vi "CalCurrent.vi"(0 "AD1":u64, 1 "AD2":u64, 2 "REAL1":dbl, 3 "REAL2":dbl, 8 "类型":u32(ring)=4 items=["PCI5121"=1, "PCI9810"=2, "USBCAN1"=3, "USBCAN2"=4, "PCI9820"=5, "CAN232"=6, "PCI5110"=7, "CANLite(mini)"=8, "ISA9620"=9, "ISA5420"=10, "PC104CAN"=11, "CANET"=17, "DNP9810"=13, "USBCAN-E-U"=20, "USBCAN-2E-U"=21], 10 "设备索引":u32(ring) items=["0", "1", "2", "3", "4", "5", "6", "7", "8", "9", "10", "11", "12", "13", "14", "15", ""], 12 "CAN路数":u32(ring) items=["0", "1"], 14 "ExternFlag":u8, 16 "ID Send":u32, 18 "DataLen":u8) -> (20 "发送状态":bool, 21 "Gain":dbl)   [LabVIEW 2013]
uses:
  BHN01/AutoBurn/Settings/ControlCAN.dll
panel:
  in  "设备索引 2":u32(ring) items=["0", "1", "2", "3", "4", "5", "6", "7", "8", "9", "10", "11", "12", "13", "14", "15", ""]
  in  "CAN路数 2":u32(ring) items=["0", "1"]
  in  "类型 2":u32(ring)=4 items=["PCI5121"=1, "PCI9810"=2, "USBCAN1"=3, "USBCAN2"=4, "PCI9820"=5, "CAN232"=6, "PCI5110"=7, "CANLite(mini)"=8, "ISA9620"=9, "ISA5420"=10, "PC104CAN"=11, "CANET"=17, "DNP9810"=13, "USBCAN-E-U"=20, "USBCAN-2E-U"=21]
  out "VCI_CAN_OBJ_T":T1 {"ID" format="%x"}
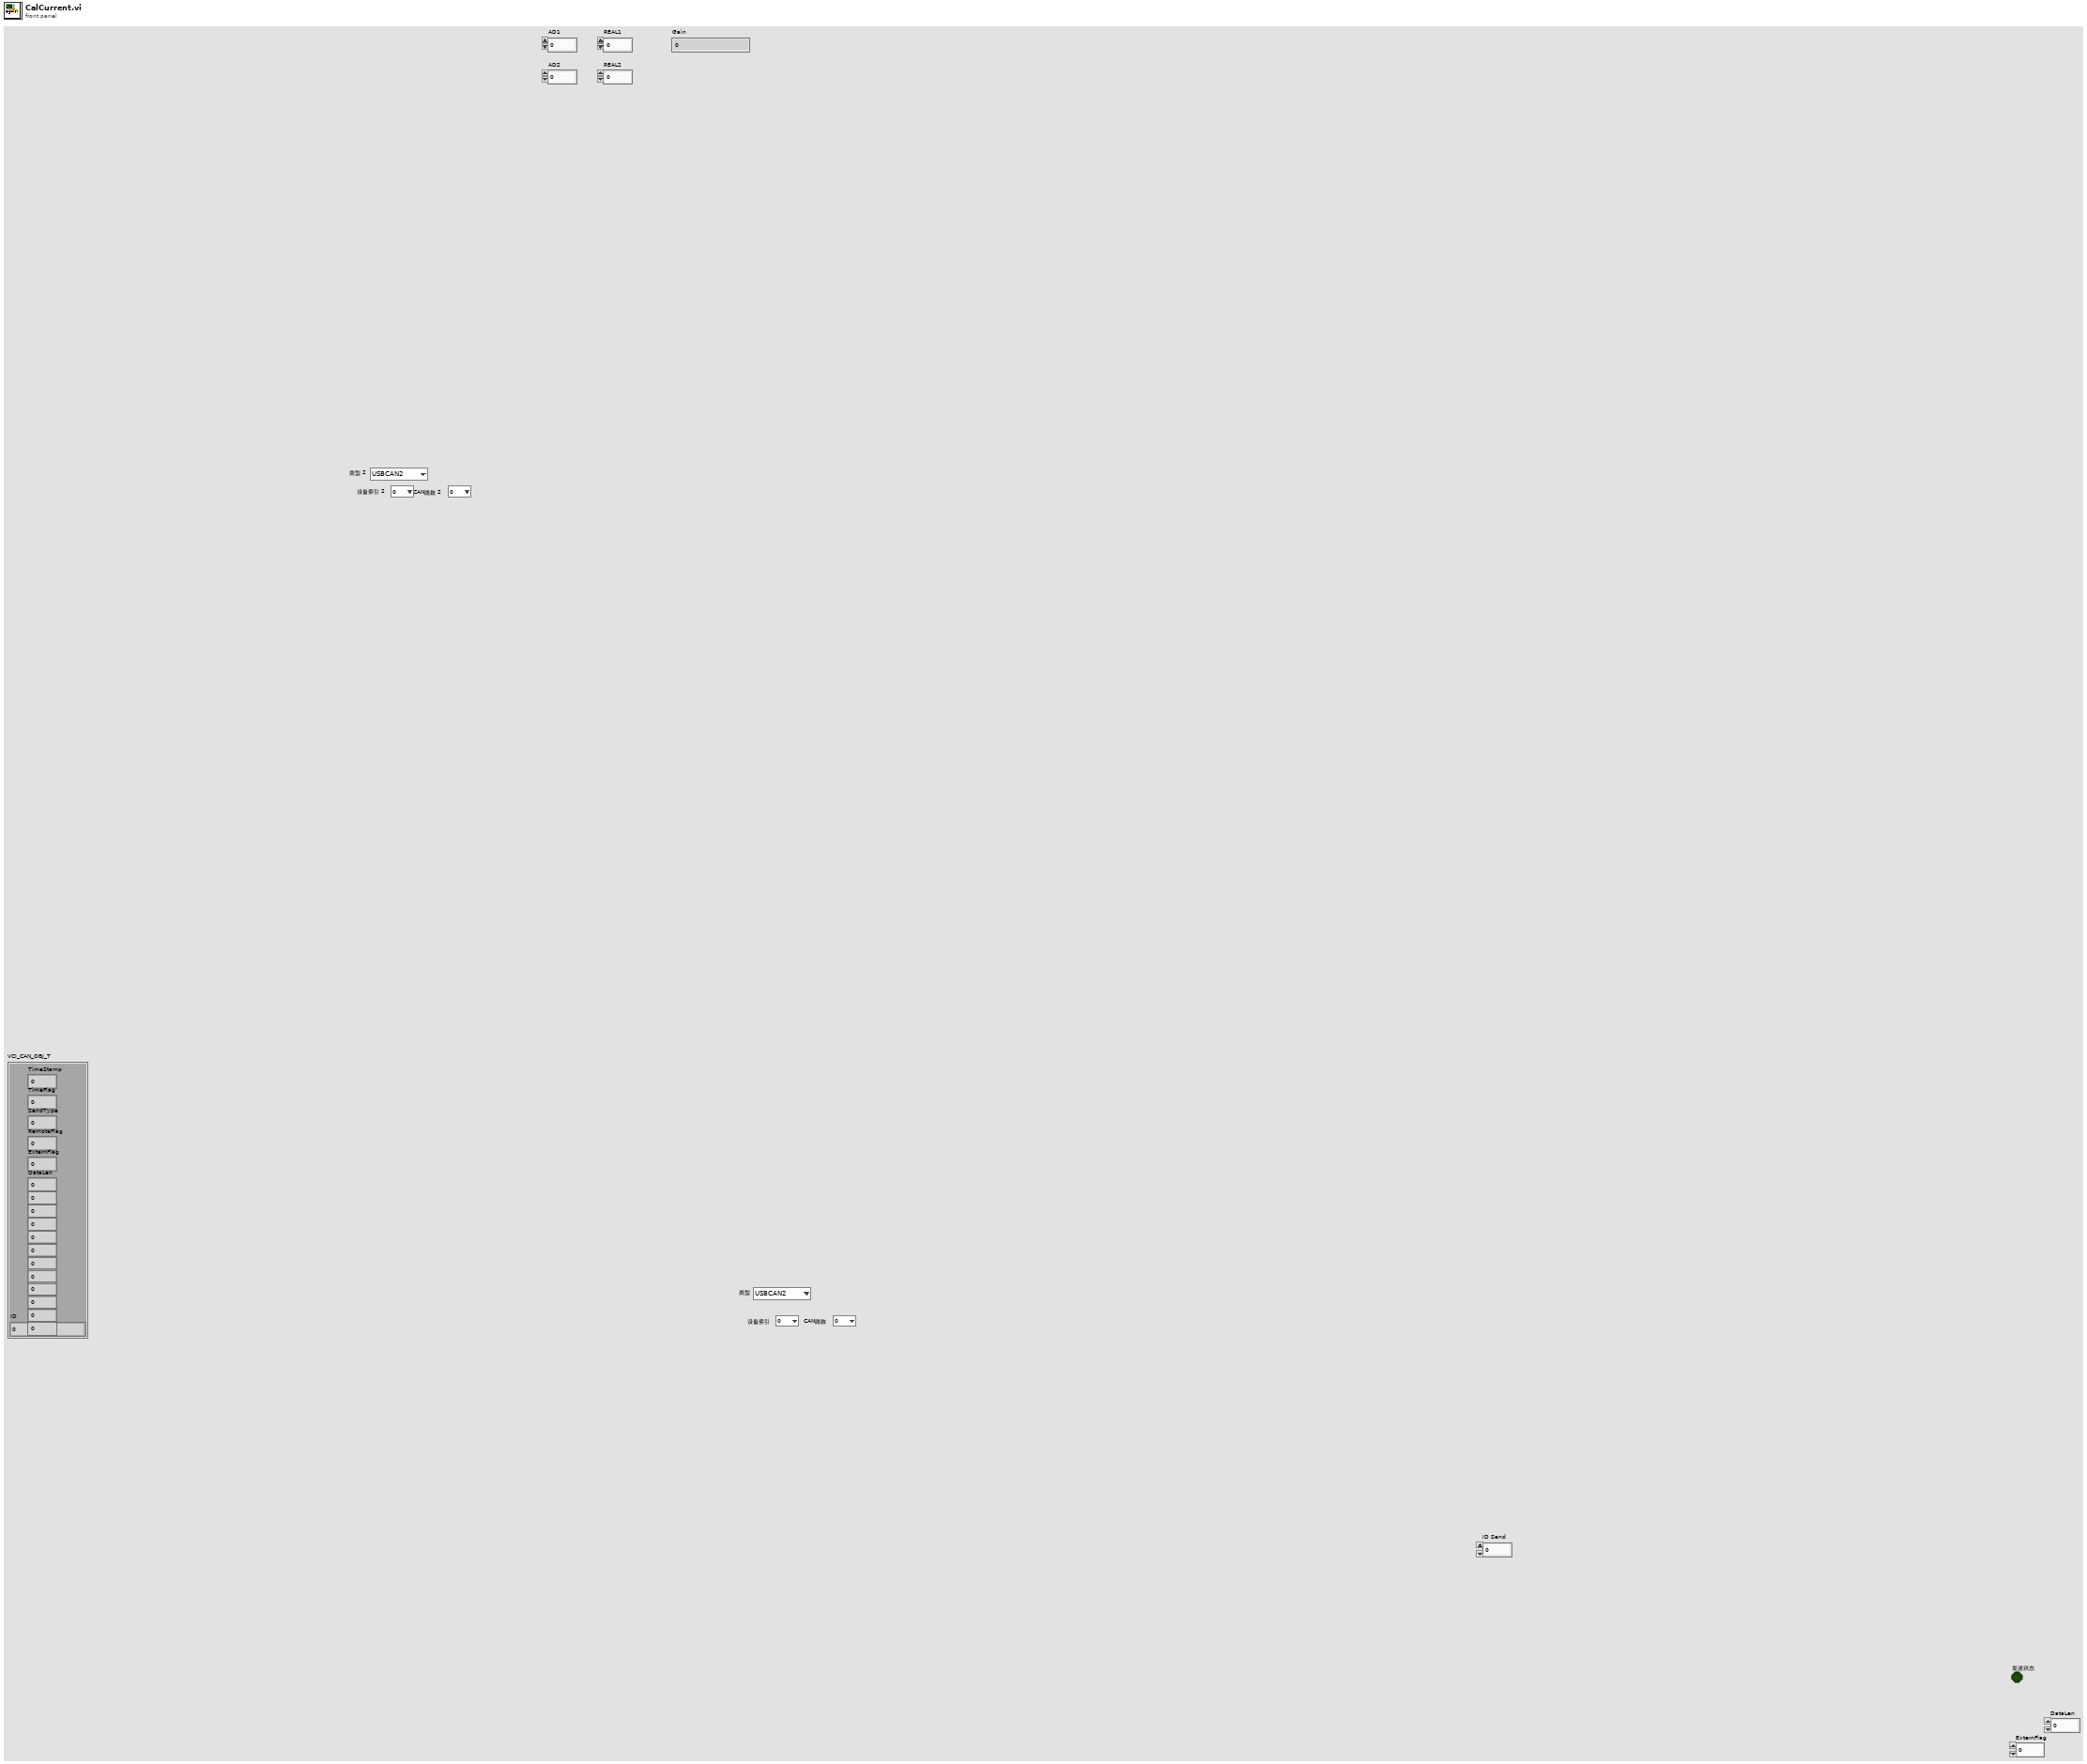
[diagram p1: front panel]
types:
  T1 = cluster{"ID":u32, "TimeStamp":u32, "TimeFlag":u8, "SendType":u8, "RemoteFlag":u8, "ExternFlag":u8, "DataLen":u8, u8, u8, u8, u8, u8, u8, u8, u8, u8, u8, u8}
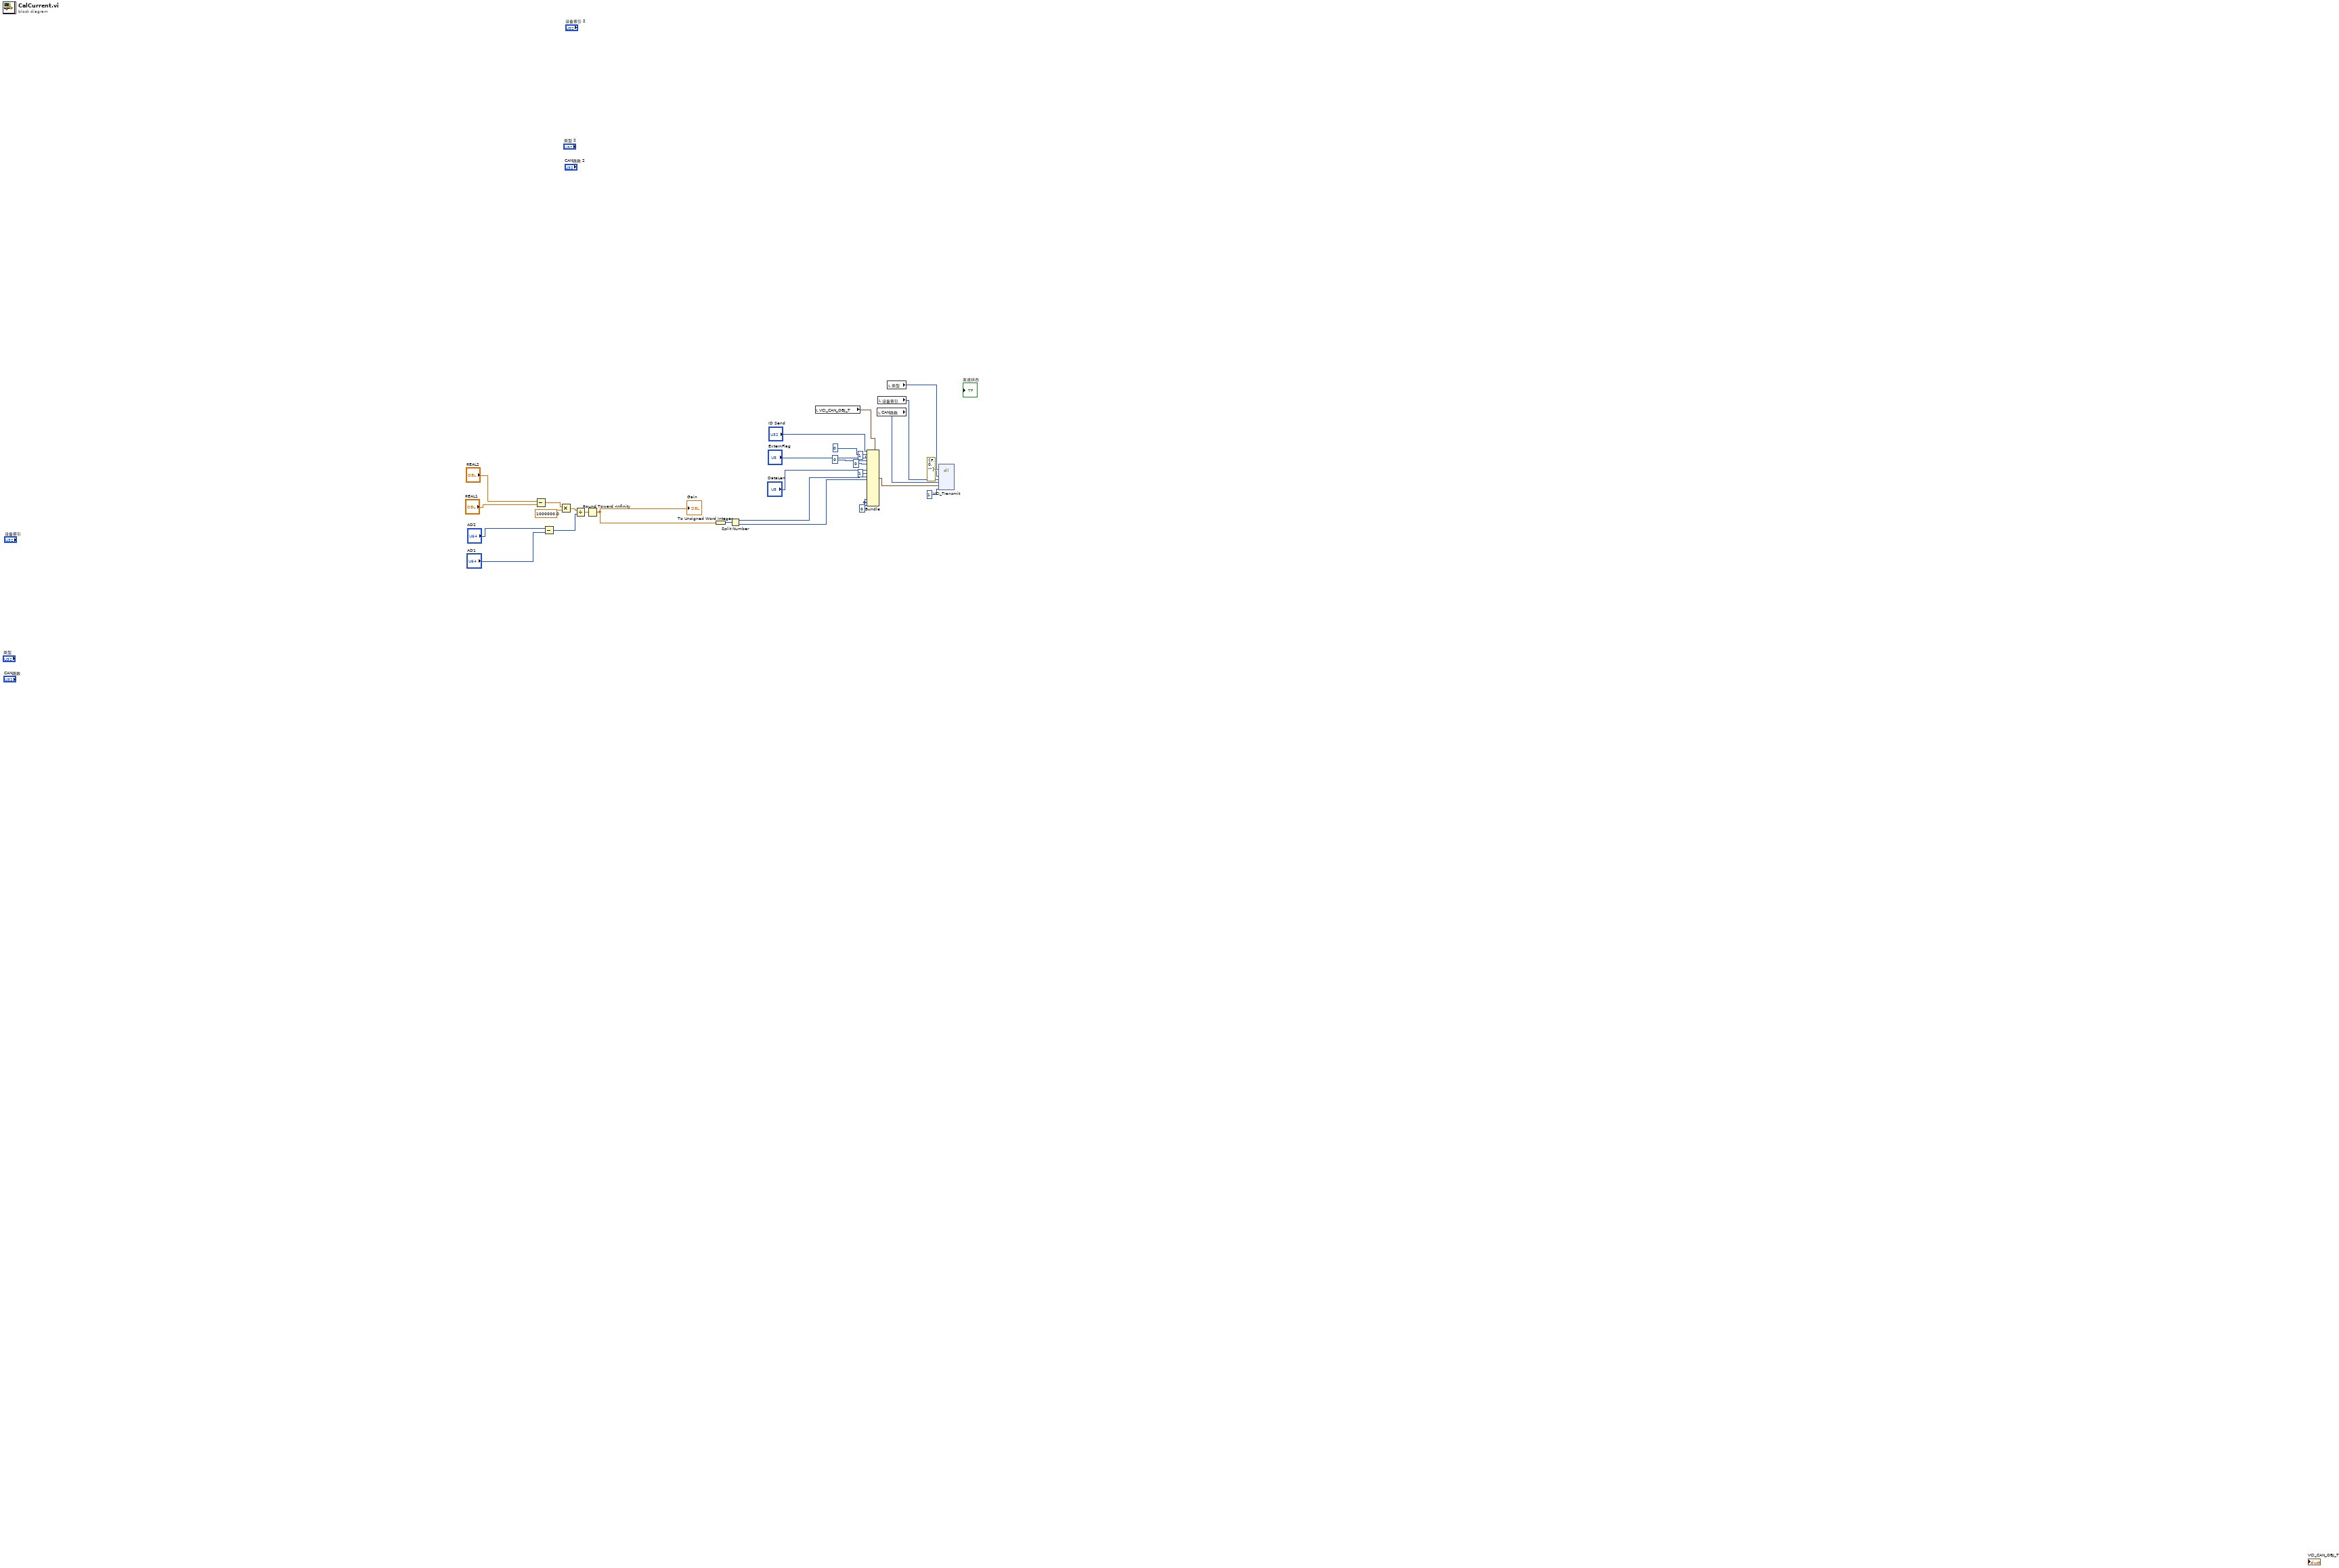
[diagram p0: block diagram]
diagram:
  w23 = u8 0 ("元素")
  n1 = Subtract(x="REAL2", y="REAL1") -> (x-y=w10:dbl)
  n2 = Subtract(x="AD2", y="AD1") -> (x-y=w8:u64)
  n3 = Multiply(x=w10, y=1000000.0) -> (x*y=w9:dbl)
  n4 = Divide(x=w9, y=w8) -> (x/y=w7:dbl)
  n5 = Round Toward -Infinity(1:w7) -> (0:w2:dbl)
  "Gain" <- w2
  n6 = To Unsigned Word Integer(number=w2) -> (unsigned 16bit integer=w14:u16)
  n7 = Split Number(x=w14) -> (hi(x)=w13:u8, lo(x)=w12:u8)
  n8 = local read "VCI_CAN_OBJ_T"() -> (w27:T1)
  n9 = Bundle(cluster=w27, "ID"="ID Send", "TimeStamp"=u8 0 ("RemoteFlag"), "TimeFlag"=u8 1, "SendType"=u8 0 ("DataLen"), "RemoteFlag"=u8 0, "ExternFlag"="ExternFlag", "DataLen"="DataLen", u8 1, w13, w12, w23, w23, w23) -> (w28:T1)  [unwired: 5 in]
  n10 = local read "CAN路数"() -> (w15:u32)
  n11 = local read "设备索引"() -> (w16:u32)
  n12 = local read "类型"() -> (w17:u32)
  n13 = dll-call lib="F:/Bluewave New Energy/SVN_Work/AutoTest_TestStand/trunk/AutoTest_TestStand/Driver/ZlgCan/BHN01/AutoBurn/Settings/ControlCAN.dll" fn="VCI_Transmit"(error in=errorcluster {"status"=FALSE, "code"=0, "source"=""} ("错误输入（无错误）"), "DeviceType"=w17, "DeviceInd"=w16, "CANInd"=w15, "pSend"=w28, "Len"=u32 1) -> ()  [unwired: 4 in, 6 out]
